vi "Chronos TDMS Get Start and End Time.vi"(8 "error in (no error)":errorcluster, 11 "file path":path) -> (0 "error out":errorcluster, 2 "end time":timestamp, 3 "Start time":timestamp)   [LabVIEW 2021]
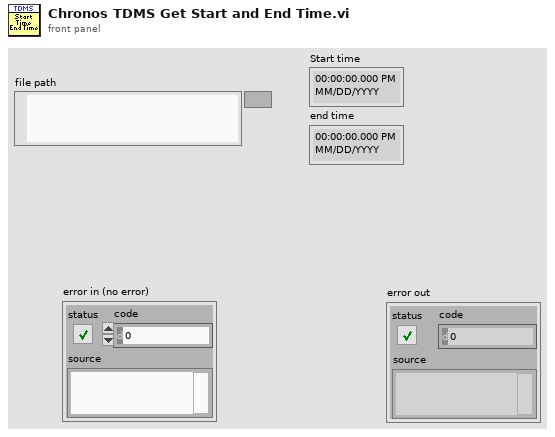
[diagram p1: front panel]
types:
  T1 = enum16{"open", "open or create", "create or replace", "create", "open (read-only)"}
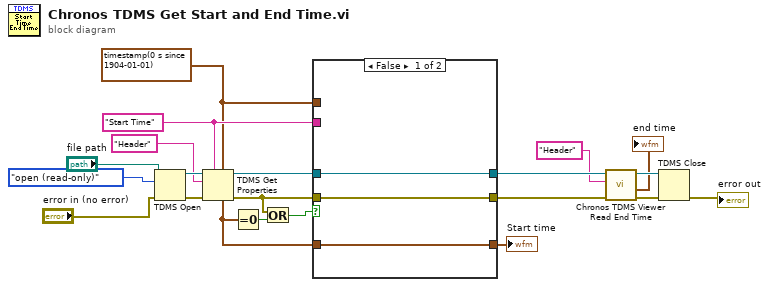
[diagram p0: block diagram]
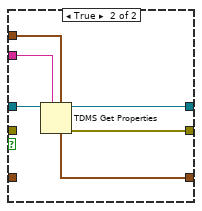
[diagram p2: hidden frame]
diagram:
  w9 = timestamp(0 s since 1904-01-01)
  w10 = "Start Time" ("group name")
  n1 = TDMS Open(8:"error in (no error)", 10:T1."open (read-only)" ("operation (0:open)"), 11:"file path") -> (0:w20:errorcluster, 3:w19:refnum<k34>)  [unwired: 4 in]
  n2 = TDMS Get Properties(5:w9, 7:w10, 8:w20, 10:"Header" ("group name"), 11:w19) -> (0:w2:errorcluster, 3:w13:refnum<k34>, 4:w1:timestamp)  [unwired: 1 in, 3 out]
  n3 = Equal To 0?(x=w1) -> (x = 0?=w4:bool)
  n4 = Or(x=w2, y=w4) -> (x .or. y?=w3:bool)
  n5 = case shown="False" w3 {
    tunnel: w13 -> [w24 w30]
    tunnel: [w24 w25] -> w12
    tunnel: [w22 w26] -> w11
    tunnel: w10 -> [_ w29]
    tunnel: w9 -> [_ w28]
    tunnel: [w23 w27] -> w8
    tunnel: w1 -> [w23 _]
    tunnel: w2 -> [w22 _]
    frame False {
    }
    frame True {
      n6 = TDMS Get Properties(5:w28, 7:w29, 11:w30) -> (0:w26:errorcluster, 3:w25:refnum<k34>, 4:w27:timestamp)  [unwired: 3 in, 3 out]
    }
  }
  "Start time" <- w8
  n7 = call "Chronos TDMS Viewer Read End Time.vi"("error in (no error)"=w11, "group name"="Header", "tdms file"=w12) -> ("error out"=w17:errorcluster, "end time"=→"end time":timestamp, "tdms file dup"=w16:refnum<k34>)  [unwired: 5 in, 1 out]
  n8 = TDMS Close(8:w17, 11:w16) -> (0:→"error out":errorcluster)  [unwired: 1 out]
